vi "File-Generator Module.vi"(11 "Metadata for all trials/volumes":T1[](array[typedef])=[{"Imaging Protocol"=enum."Functional Acquisition", "Number of Trials"=2, "Frame Size"=512, "# Averaged frames"=1, "Dwell time (us)"=0.1, "Index of Z-plane"=0, "Timelapse?"=FALSE, "Logging process is active"=TRUE, "Speed logging enabled"=FALSE, "tdms file ref"=refnum, "path"=path "E:/UCL/Rig 3 MovCor integration version/Datasets/Dual Plane datasets/150701_01_13_28/Functional imaging TDMS data files/001.tdms", "Trial Number"=1, "Expected # points acquired"=TRUE, "Manually stopped"=FALSE, "Ch0 data"=[], "Ch1 data"=[], "Last trial"=FALSE, "Points acquired"={"Ch0 last trial"=0, "Ch1 last trial"=0, "All trials"=0}}, {"Imaging Protocol"=enum."Functional Acquisition", "Number of Trials"=2, "Frame Size"=512, "# Averaged frames"=1, "Dwell time (us)"=0.1, "Index of Z-plane"=0, "Timelapse?"=FALSE, "Logging process is active"=TRUE, "Speed logging enabled"=FALSE, "tdms file ref"=refnum, "path"=path "E:/UCL/Rig 3 MovCor integration version/Datasets/Dual Plane datasets/150701_01_13_28/Functional imaging TDMS data files/002.tdms", "Trial Number"=2, "Expected # points acquired"=TRUE, "Manually stopped"=FALSE, "Ch0 data"=[], "Ch1 data"=[], "Last trial"=FALSE, "Points acquired"={"Ch0 last trial"=0, "Ch1 last trial"=0, "All trials"=0}}, {"Imaging Protocol"=enum."Functional Acquisition", "Number of Trials"=2, "Frame Size"=512, "# Averaged frames"=1, "Dwell time (us)"=0.1, "Index of Z-plane"=0, "Timelapse?"=FALSE, "Logging process is active"=TRUE, "Speed logging enabled"=FALSE, "tdms file ref"=refnum, "path"=path "E:/UCL/Rig 3 MovCor integration version/Datasets/Dual Plane datasets/150701_01_13_28/Functional imaging TDMS data files/003.tdms", "Trial Number"=2, "Expected # points acquired"=TRUE, "Manually stopped"=FALSE, "Ch0 data"=[], "Ch1 data"=[], "Last trial"=FALSE, "Points acquired"={"Ch0 last trial"=0, "Ch1 last trial"=0, "All trials"=0}}] {"Frame Size" items=["100X100"=100, "128X128"=128, "200X200"=200, "256X256"=256, "512X512"=512, "1024x1024"=1024, "2048x2048"=2048]; "Dwell time (us)" format="%#.6g"}) -> ()   [LabVIEW 2013]
uses:
  Typedefs/Logging queue element.ctl
  Typedefs/Imaging Protocols enum.ctl
  Typedefs/Frame Size.ctl
  Typedefs/Acquired points count.ctl
  Typedefs/Top level VI states.ctl
  Global Variables/General Globals.vi
  Global Variables/gl_Queues.vi
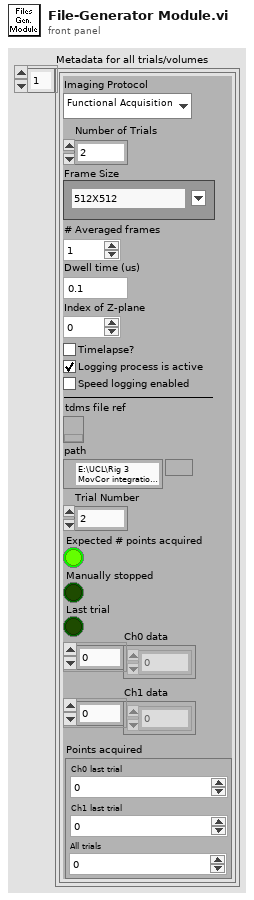
[diagram p1: front panel]
types:
  T1 = typedef "Logging queue element.ctl" = cluster{"Imaging Protocol":T2, "Number of Trials":u16, "Frame Size":T3, "# Averaged frames":u16, "Dwell time (us)":dbl, "Index of Z-plane":i32, "Timelapse?":bool, "Logging process is active":bool, "Speed logging enabled":bool, "tdms file ref":refnum<k34>, "path":path, "Trial Number":i32, "Expected # points acquired":bool, "Manually stopped":bool, "Ch0 data":u32[], "Ch1 data":u32[], "Last trial":bool, "Points acquired":T4}
  T2 = typedef "Imaging Protocols enum.ctl" = enum16{"AOL Z-Stack", "Motor Z Stack", "Functional Acquisition", "Single Plane Acquisition", "Volume Acquisition", "Live Imaging", "Live Plane Imaging", "Live Volume Imaging"}
  T3 = typedef "Frame Size.ctl" = u16
  T4 = typedef "Acquired points count.ctl" = cluster{"Ch0 last trial":u64, "Ch1 last trial":u64, "All trials":u64}
  T5 = typedef "Top level VI states.ctl" = enum16{"None", "Initialise UI", "<STACK PROTOCOL STATES>", "AOL Zstack-START", "AOL Zstack-STOP", "Motor Zstack-START", "Motor Zstack-STOP", "<ACQUISITION PROTOCOL STATES> ", "Functional Acquisition-START", "Functional Acquisition-STOP", "Single Plane Acquisition-START", "Single Plane Acquisition-STOP", "Volume Acquisition-START", "Volume Acquisition-STOP", "<LIVE IMAGING PROTOCOL STATES>", "Live Imaging-START", "Live Imaging-STOP", "Live Plane Imaging-START", "Live Plane Imaging-STOP", "Live Volume Imaging-START", "Live Volume Imaging-STOP", "EXIT"}
  T6 = typedef "All Message Queues.ctl" = cluster{"UI queue":refnum<queue>, "Acq. queue":refnum<queue>, "Logging queue":refnum<queue>}
  T7 = typedef "ROI ID Enum.ctl" = enum16{"Point", "MiniScan", "Comp. MiniScan", "Rectangle", "Comp. volume", "Arb. plane point"}
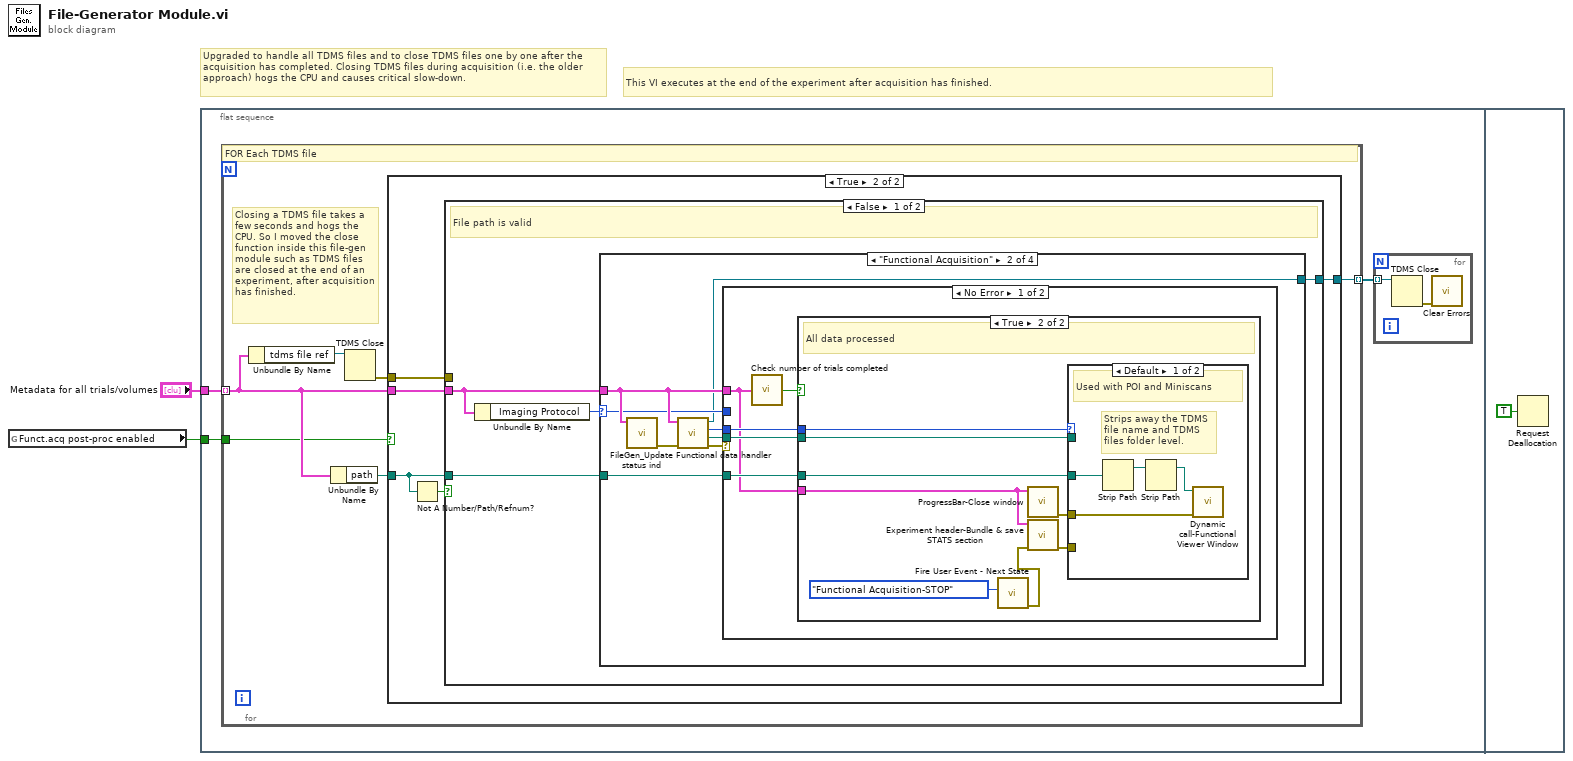
[diagram p0: block diagram]
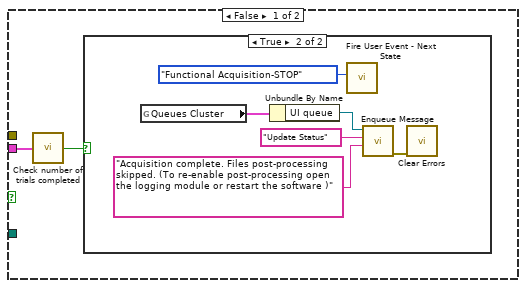
[diagram p2: hidden frame]
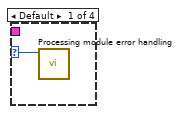
[diagram p4: hidden frame]
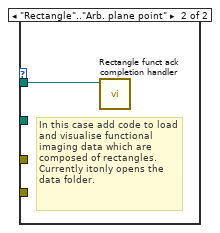
[diagram p6: hidden frame]
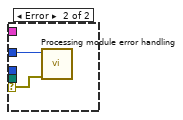
[diagram p7: hidden frame]
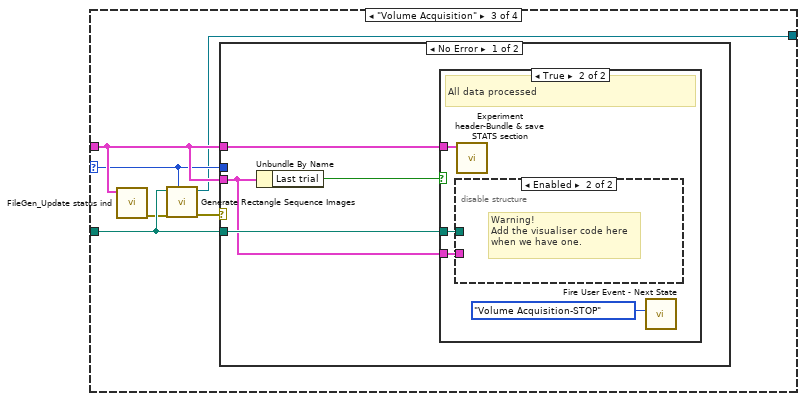
[diagram p8: hidden frame]
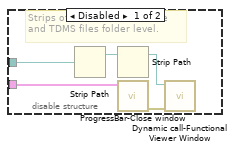
[diagram p10: hidden frame]
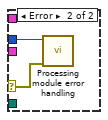
[diagram p11: hidden frame]
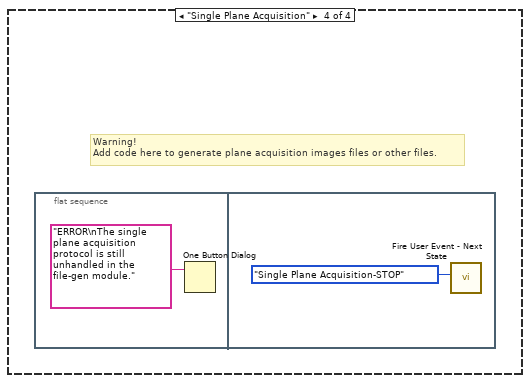
[diagram p12: hidden frame]
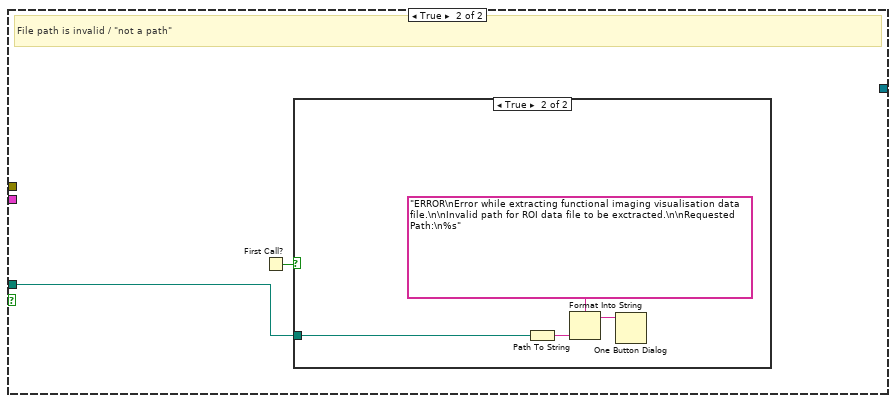
[diagram p13: hidden frame]
diagram:
  # "This VI executes at the end of the experiment after acquisition has finished."
  # "Upgraded to handle all TDMS files and to close TDMS files one by one after the acquisition has completed. Closing TDMS files during acquisition (i.e. the older approach) hogs the CPU and causes critical slow-down."
  n1 = global read "General Globals.vi" "Funct.acq post-proc enabled"() -> (w1:bool)
  n2 = flat-sequence {
    tunnel: "Metadata for all trials/volumes" -> [w5]
    tunnel: w1 -> [w4]
    frame #0 {
      n3 = for {
        tunnel: w5 -> [w11] mode=indexing
        tunnel: w4 -> [w9]
        tunnel: [w8] -> w3 mode=indexing
        # "Closing a TDMS file takes a few seconds and hogs the CPU. So I moved the close function inside this file-gen module such as TDMS files are closed at the end of an experiment, after acquisition has finished."
        # "FOR Each TDMS file"
        n4 = Unbundle By Name(w11) -> ("tdms file ref"=w12:refnum<k34>)
        n5 = Unbundle By Name(w11) -> ("path"=w13:path)
        n6 = TDMS Close(11:w12) -> (0:w10:errorcluster)  [unwired: 1 in, 1 out]
        n7 = case shown="True" w9 {
          tunnel: w13 -> [_ w26]
          tunnel: w11 -> [w15 w25]
          tunnel: w10 -> [_ w24]
          tunnel: [_ w22] -> w8
          frame False {
            n8 = call "Check number of trials completed.vi"("Cluster"=w15) -> ("# of trials completed"=w14:bool)
            n9 = case shown="True" w14 {
              frame False {
              }
              frame True {
                n10 = global read "gl_Queues.vi" "Queues Cluster"() -> (w19:T6)
                n11 = Unbundle By Name(w19) -> ("UI queue"=w18:refnum<queue>)
                n12 = call "Fire User Event - Next State.vi"("\"UI Handler loop\" case to execute"=Top_level_VI_states."Functional Acquisition-STOP" ("event data / imaging mode")) -> ()  [unwired: 10 in, 1 out]
                n13 = call "Enqueue Message.vi"("Message Data"="Acquisition complete. Files post-processing skipped. (To re-enable post-processing open the logging module or restart the software )" ("Acquiring and Logging..."), "Message"="Update Status", "Queue"=w18) -> ("error out"=w17:errorcluster)  [unwired: 7 in, 1 out]
                n14 = call <vilib>:"Clear Errors.vi"("error in (no error)"=w17) -> ()  [unwired: 6 in, 1 out]
              }
            }
          }
          frame True {
            n15 = Not A Number/Path/Refnum?(number/path/refnum=w26) -> (NaN/Path/Refnum?=w23:bool)
            n16 = case shown="False" w23 {
              tunnel: w26 -> [w30 w84]
              tunnel: w25 -> [w28 _]
              tunnel: w24 -> [_ _]
              tunnel: [w27 _] -> w22
              frame False {
                # "File path is valid"
                n17 = Unbundle By Name(w28) -> ("Imaging Protocol"=w29:T2)
                n18 = case shown="\"Functional Acquisition\"" w29 {
                  selector: w29 -> [w31 w33 w61 _]
                  tunnel: w28 -> [_ w34 w62 _]
                  tunnel: w30 -> [_ w38 w65 _]
                  tunnel: [_ w32 w60 _] -> w27
                  frame Default {
                    n19 = call "Processing module error handling.vi"("Imaging Protocol"=w31) -> ()  [unwired: 11 in]
                  }
                  frame "Functional Acquisition" {
                    n20 = call "FileGen_Update status ind.vi"("Cluster"=w34) -> ("error out"=w35:errorcluster)  [unwired: 10 in]
                    n21 = call "Functional data handler.vi"("error in"=w35, "Setup cluster"=w34) -> ("error out"=w39:errorcluster, "Destination fiolder"=w36:path, "Predominant ROI type"=w37:T7, "tdms file to close"=w32:refnum<k34>)  [unwired: 6 in]
                    n22 = case shown="No Error" w39 {
                      selector: w39 -> [_ w59]
                      tunnel: w38 -> [w43 _]
                      tunnel: w34 -> [w40 _]
                      tunnel: w37 -> [w42 _]
                      tunnel: w36 -> [w41 _]
                      tunnel: w33 -> [_ w58]
                      frame No Error {
                        n23 = call "Check number of trials completed.vi"("Cluster"=w40) -> ("# of trials completed"=w44:bool)
                        n24 = case shown="True" w44 {
                          tunnel: w43 -> [_ w52]
                          tunnel: w40 -> [_ w48]
                          tunnel: w42 -> [_ w50]
                          tunnel: w41 -> [_ w49]
                          frame False {
                            # "Still processing..."
                          }
                          frame True {
                            # "All data processed"
                            n25 = call "Fire User Event - Next State.vi"("\"UI Handler loop\" case to execute"=Top_level_VI_states."Functional Acquisition-STOP" ("event data / imaging mode")) -> ("Error Out"=w45:errorcluster)  [unwired: 10 in]
                            n26 = call "ProgressBar-Close window.vi"("Z-stack queue cluster"=w48) -> ("error out (no error)"=w51:errorcluster)  [unwired: 10 in]
                            n27 = call "Experiment header-Bundle & save STATS section.vi"("error in (no error)"=w45, "Logging queue element"=w48) -> ("error out"=w47:errorcluster)  [unwired: 9 in]
                            n28 = case shown="Default" w50 {
                              tunnel: w52 -> [w55 _]
                              tunnel: w51 -> [w54 _]
                              tunnel: w49 -> [_ w57]
                              tunnel: w47 -> [_ _]
                              frame Default {
                                # "Strips away the TDMS file name and TDMS files folder level."
                                # "Used with POI and Miniscans"
                                n29 = Strip Path(path=w55) -> (stripped path=w56:path)  [unwired: 1 out]
                                n30 = Strip Path(path=w56) -> (stripped path=w53:path)  [unwired: 1 out]
                                n31 = call "Dynamic call-Functional Viewer Window.vi"("error in (no error)"=w54, "Experiment data folder path"=w53) -> ()  [unwired: 10 in]
                              }
                              frame "Rectangle".."Arb. plane point" {
                                # "In this case add code to load and visualise functional imaging data which are composed of rectangles.\nCurrently itonly opens the data folder."
                                n32 = call "Rectangle funct ack completion handler.vi"("Destination fiolder"=w57) -> ()  [unwired: 11 in]
                              }
                            }
                          }
                        }
                      }
                      frame Error {
                        n33 = call "Processing module error handling.vi"("error in (no error)"=w59, "Imaging Protocol"=w58) -> ()  [unwired: 10 in]
                      }
                    }
                  }
                  frame "Volume Acquisition" {
                    n34 = call "FileGen_Update status ind.vi"("Cluster"=w62) -> ("error out"=w63:errorcluster)  [unwired: 10 in]
                    n35 = call "Generate Rectangle Sequence Images.vi"("Imaging Protocol"=w61, "error in (no error)"=w63, "TDMS file path & name"=w65) -> ("error out"=w64:errorcluster, "tdms file to close"=w60:refnum<k34>)  [unwired: 6 in, 1 out]
                    n36 = case shown="No Error" w64 {
                      selector: w64 -> [_ w80]
                      tunnel: w65 -> [w69 _]
                      tunnel: w62 -> [w68 _]
                      tunnel: w62 -> [w66 _]
                      tunnel: w61 -> [_ w79]
                      frame No Error {
                        n37 = Unbundle By Name(w68) -> ("Last trial"=w67:bool)
                        n38 = case shown="True" w67 {
                          tunnel: w69 -> [_ w73]
                          tunnel: w68 -> [_ w72]
                          tunnel: w66 -> [_ w70]
                          frame False {
                            # "Still processing..."
                          }
                          frame True {
                            # "All data processed"
                            n39 = disable-structure shown="Enabled" {
                              disable-tunnel: w73 -> [w77 _]
                              disable-tunnel: w72 -> [w76 _]
                              frame Disabled {
                                # "Strips off the TDMS file name and TDMS files folder level."
                                n40 = Strip Path(path=w77) -> (stripped path=w78:path)  [unwired: 1 out]
                                n41 = Strip Path(path=w78) -> (stripped path=w74:path)  [unwired: 1 out]
                                n42 = call "ProgressBar-Close window.vi"("Z-stack queue cluster"=w76) -> ("error out (no error)"=w75:errorcluster)  [unwired: 10 in]
                                n43 = call "Dynamic call-Functional Viewer Window.vi"("error in (no error)"=w75, "Experiment data folder path"=w74) -> ()  [unwired: 10 in]
                              }
                              frame Enabled {
                                # "Warning!\nAdd the visualiser code here\nwhen we have one."
                              }
                            }
                            n44 = call "Experiment header-Bundle & save STATS section.vi"("Logging queue element"=w70) -> ()  [unwired: 10 in, 1 out]
                            n45 = call "Fire User Event - Next State.vi"("\"UI Handler loop\" case to execute"=Top_level_VI_states."Volume Acquisition-STOP" ("event data / imaging mode")) -> ()  [unwired: 10 in, 1 out]
                          }
                        }
                      }
                      frame Error {
                        n46 = call "Processing module error handling.vi"("error in (no error)"=w80, "Imaging Protocol"=w79) -> ()  [unwired: 10 in]
                      }
                    }
                  }
                  frame "Single Plane Acquisition" {
                    # "Warning!\nAdd code here to generate plane acquisition images files or other files."
                    n47 = flat-sequence {
                      frame #0 {
                        n48 = One Button Dialog(message="ERROR\nThe single plane acquisition protocol is still unhandled in the file-gen module.") -> ()  [unwired: 1 in, 1 out]
                      }
                      frame #1 {
                        n49 = call "Fire User Event - Next State.vi"("\"UI Handler loop\" case to execute"=Top_level_VI_states."Single Plane Acquisition-STOP" ("event data / imaging mode")) -> ()  [unwired: 10 in, 1 out]
                      }
                    }
                  }
                }
              }
              frame True {
                # "File path is invalid / \"not a path\""
                n50 = First Call?() -> (First Call?: T/F=w83:bool)
                n51 = case shown="True" w83 {
                  tunnel: w84 -> [_ w88]
                  frame False {
                  }
                  frame True {
                    n52 = Path To String(path=w88) -> (string=w86:string)
                    n53 = Format Into String(format string="ERROR\nError while extracting functional imaging visualisation data file.\n\nInvalid path for ROI data file to be exctracted.\n\nRequested Path:\n%s", w86) -> (resulting string=w85:string)  [unwired: 2 in, 1 out]
                    n54 = One Button Dialog(message=w85) -> ()  [unwired: 1 in, 1 out]
                  }
                }
              }
            }
          }
        }
      }
      n55 = for {
        tunnel: w3 -> [w7] mode=indexing
        n56 = TDMS Close(11:w7) -> (0:w6:errorcluster)  [unwired: 1 in, 1 out]
        n57 = call <vilib>:"Clear Errors.vi"("error in (no error)"=w6) -> ()  [unwired: 6 in, 1 out]
      }
    }
    frame #1 {
      n58 = Request Deallocation(TRUE ("flag")) -> ()
    }
  }
